vi "LogicTrain-Sample-05-01-ALT.vi"() -> ()   [LabVIEW 2020]
uses:
  <vilib>/Rock Robotics/WPI/ThirdParty/JAS_Junk/TrajLib/Timer_New.vi
  <vilib>/Utility/semaphor.llb/Obtain Semaphore Reference.vi
  <vilib>/Rock Robotics/WPI/ThirdParty/JAS_Junk/TrajLib/Timer_Reset.vi
  <vilib>/Rock Robotics/WPI/ThirdParty/JAS_Junk/TrajLib/Timer_Start.vi
  <vilib>/Rock Robotics/WPI/ThirdParty/JAS_Junk/TrajLib/Timer_Stop.vi
  <vilib>/Rock Robotics/WPI/ThirdParty/JAS_Junk/TrajLib/Timer_HasPeriodPassedOnce.vi
  <vilib>/Rock Robotics/WPI/ThirdParty/JAS_Junk/TrajLib/Trajectory_Library.lvlib
panel:
  out "Ready":bool
  out "Extend Arm":bool
  out "Close Hand":bool
  in  "Capture Cube":bool
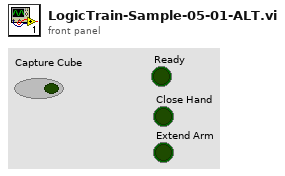
[diagram p1: front panel]
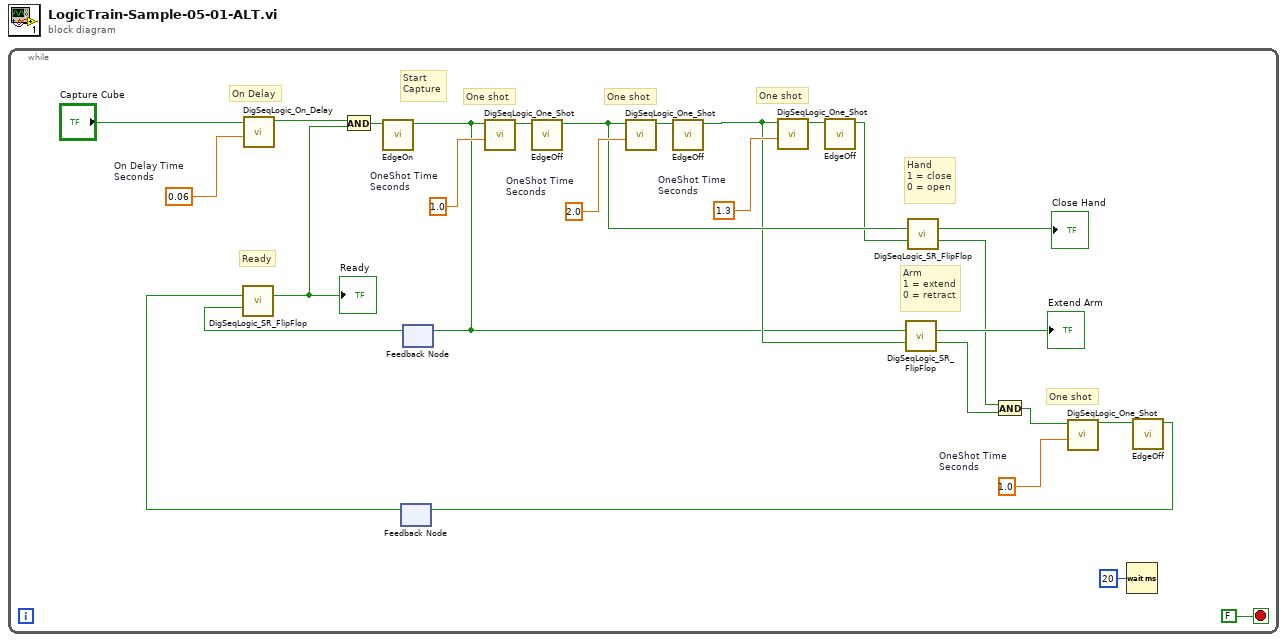
[diagram p0: block diagram]
diagram:
  n1 = while {
    stop <- FALSE stop-if-true
    w18 = 1.3  # OneShot Time Seconds
    w20 = 2.0  # OneShot Time Seconds
    w23 = 1.0  # OneShot Time Seconds
    w26 = 0.06  # On Delay Time Seconds
    w27 = 1.0  # OneShot Time Seconds
    # "Ready"
    # "Arm\n1 = extend\n0 = retract"
    # "Hand\n1 = close\n0 = open"
    # "One shot"
    # "One shot"
    # "Start\nCapture"
    # "One shot"
    # "On Delay"
    # "One shot"
    n2 = call <vilib>:"DigSeqLogic_On_Delay.vi"("Delay"=w26, "Input"="Capture Cube") -> ("Output"=w24:bool)  [unwired: 8 in, 1 out]
    n3 = feedback #1() -> (w5:bool)  [unwired: 1 in]
    n4 = feedback #2() -> (w3:bool)  [unwired: 1 in]
    n5 = call <vilib>:"DigSeqLogic_SR_FlipFlop.vi"("Set"=w5, "Reset"=w3) -> ("Output"=w11:bool)  [unwired: 12 in, 1 out]
    "Ready" <- w11
    n6 = And(x=w24, y=w11) -> (x .and. y?=w22:bool)
    n7 = call "EdgeOn.vi"("Input"=w22) -> ("Edge On"=w4:bool)  [unwired: 10 in]
    n8 = feedback-in #2(w4) -> ()
    n9 = call <vilib>:"DigSeqLogic_One_Shot.vi"("OneShot"=w23, "Input"=w4) -> ("Output"=w21:bool)  [unwired: 8 in, 1 out]
    n10 = call "EdgeOff.vi"("Input"=w21) -> ("Edge Off"=w16:bool)  [unwired: 10 in]
    n11 = call <vilib>:"DigSeqLogic_One_Shot.vi"("OneShot"=w20, "Input"=w16) -> ("Output"=w19:bool)  [unwired: 8 in, 1 out]
    n12 = call "EdgeOff.vi"("Input"=w19) -> ("Edge Off"=w15:bool)  [unwired: 10 in]
    n13 = call <vilib>:"DigSeqLogic_One_Shot.vi"("OneShot"=w18, "Input"=w15) -> ("Output"=w17:bool)  [unwired: 8 in, 1 out]
    n14 = call "EdgeOff.vi"("Input"=w17) -> ("Edge Off"=w14:bool)  [unwired: 10 in]
    n15 = call <vilib>:"DigSeqLogic_SR_FlipFlop.vi"("Set"=w4, "Reset"=w15) -> ("Output"=→"Extend Arm":bool, "Inverse Output"=w9:bool)  [unwired: 12 in]
    n16 = call <vilib>:"DigSeqLogic_SR_FlipFlop.vi"("Set"=w16, "Reset"=w14) -> ("Output"=→"Close Hand":bool, "Inverse Output"=w10:bool)  [unwired: 12 in]
    n17 = And(x=w10, y=w9) -> (x .and. y?=w8:bool)
    n18 = call <vilib>:"DigSeqLogic_One_Shot.vi"("OneShot"=w27, "Input"=w8) -> ("Output"=w7:bool)  [unwired: 8 in, 1 out]
    n19 = Wait (ms)(milliseconds to wait=u32 20) -> ()  [unwired: 1 out]
    n20 = call "EdgeOff.vi"("Input"=w7) -> ("Edge Off"=w6:bool)  [unwired: 10 in]
    n21 = feedback-in #1(w6) -> ()
  }
